vi "xxxx.vi"(8 "error in (no error)":errorcluster, 11 "xxxx in":refnum<class "xxxx.lvclass">) -> (0 "error out":errorcluster, 3 "xxxx out":refnum<class "xxxx.lvclass">)   [LabVIEW 2021, in "xxxx.lvlib" / "xxxx.lvclass"]
uses:
  xxxx.lvclass
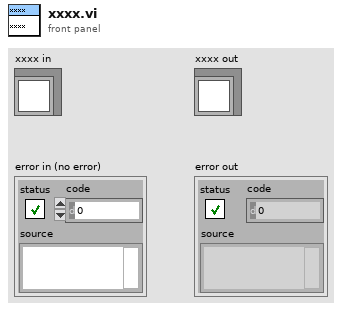
[diagram p1: front panel]
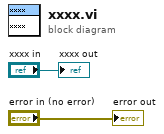
[diagram p0: block diagram]
diagram:
  "error out" <- "error in (no error)"
  "xxxx out" <- "xxxx in"
